vi "Acquire Every Image as Raw Data.vi"() -> ()   [LabVIEW 2023]
doc: "The Acquire Every Image as Raw Data example acquires images continuously and returns an array of the pixel data. This functionality can be useful for getting access to the raw data to stream it to disk in a binary format or pass it to a third-party processing function."
uses:
  <vilib>/vision/driver/IMAQdx.llb/IMAQdx Buffer Number Mode.ctl
  <vilib>/vision/driver/NI_Vision_Acquisition_Software.lvlib
  <resource>/objmgr/imaqdx.rc
panel:
  in  "Percent of Images Reserved by Driver":dbl=50.0
  in  "Overwrite Mode":u16(ring) items=["Get Oldest"=0, "Fail"=2, "Get Newest"=3]
  in  "Number of Images":i32=10
  out "Image Data Size (bytes)":i32
  out "Image Data":u8[](array[numeric])
  in  "Simulated Processing Delay (ms)":i32
  out "Images Missed":u32
  out "Images Behind":i32
  out "Processing Frame Rate":dbl
  in  "Camera Name":refnum<k21> caption="IMAQdx Session"
  out "Buffer Number":u32
  out "Acquired Frame Rate":dbl
  in  "Stop":bool
  # "Overview: Demonstrates how to acquire the raw data from a camera, which may be useful for streaming to disk or passing to third-party party image processing functions.\nRequirements: Vision Acquisition Software\nInstructions:\n1. Select the Camera Name\n2. Run the VI\n3. Increase the Simulated Processing Delay to see the effect on Images Behind and Images Missed when the acquisition loop isn't executed as quickly as the camera acquires images."
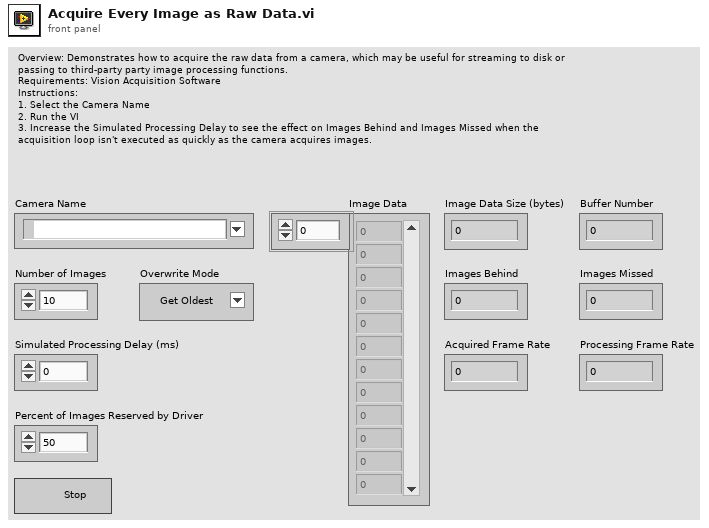
[diagram p1: front panel]
types:
  T1 = typedef "IMAQdx.ctl" = refnum<k21>
  T2 = typedef "NI_Vision_Acquisition_Software.lvlib/IMAQdx Buffer Number Mode.ctl" = enum32{"Next", "Last", "Buffer Number", "Every", "Last New"}
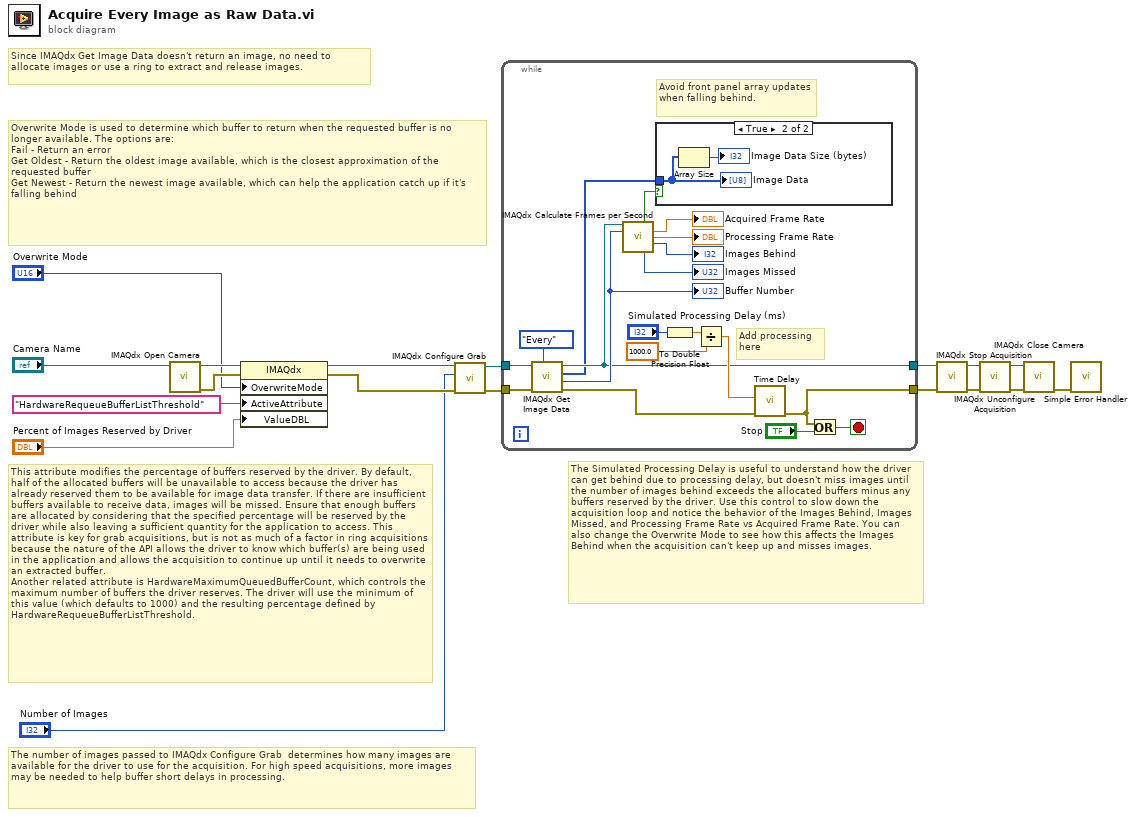
[diagram p0: block diagram]
diagram:
  # "The number of images passed to IMAQdx Configure Grab  determines how many images are available for the driver to use for the acquisition. For high speed acquisitions, more images may be needed to help buffer short delays in processing."
  # "This attribute modifies the percentage of buffers reserved by the driver. By default, half of the allocated buffers will be unavailable to access because the driver has already reserved them to be available for image data transfer. If there are insufficient buffers available to receive data, images will be missed. Ensure that enough buffers are allocated by considering that the specified percentage will be reserved by the driver while also leaving a sufficient quantity for the application to access. This attribute is key for grab acquisitions, but is not as much of a factor in ring acquisitions because the nature of the API allows the driver to know which buffer(s) are being used in the application and allows the acquisition to continue up until it needs to overwrite an extracted buffer.\nAnother related attribute is HardwareMaximumQueuedBufferCount, which controls the maximum number of buffers the driver reserves. The driver will use the minimum of this value (which defaults to 1000) and the resulting percentage defined by HardwareRequeueBufferListThreshold."
  # "The Simulated Processing Delay is useful to understand how the driver can get behind due to processing delay, but doesn't miss images until the number of images behind exceeds the allocated buffers minus any buffers reserved by the driver. Use this control to slow down the acquisition loop and notice the behavior of the Images Behind, Images Missed, and Processing Frame Rate vs Acquired Frame Rate. You can also change the Overwrite Mode to see how this affects the Images Behind when the acquisition can't keep up and misses images."
  # "Overwrite Mode is used to determine which buffer to return when the requested buffer is no longer available. The options are:\nFail - Return an error\nGet Oldest - Return the oldest image available, which is the closest approximation of the requested buffer\nGet Newest - Return the newest image available, which can help the application catch up if it's falling behind"
  # "Since IMAQdx Get Image Data doesn't return an image, no need to allocate images or use a ring to extract and release images."
  n1 = call <vilib>:"IMAQdx Open Camera.vi"("Session In"="Camera Name") -> ("error out"=w9:errorcluster, "Session Out"=w10:T1)  [unwired: 2 in, 7 out]
  n2 = property class="IMAQdx"(reference=w10, error in=w9, "OverwriteMode"="Overwrite Mode", "ActiveAttribute"="HardwareRequeueBufferListThreshold", "ValueDBL"="Percent of Images Reserved by Driver") -> (reference out=w8:T1, error out=w7:errorcluster)
  n3 = call <vilib>:"IMAQdx Configure Grab.vi"("error in"=w7, "Number of Buffers"="Number of Images", "Session In"=w8) -> ("error out"=w5:errorcluster, "Session Out"=w6:T1)  [unwired: 7 in]
  n4 = while {
    tunnel: [w24] -> w13
    tunnel: w5 -> [w27]
    tunnel: w6 -> [w28]
    tunnel: [w33] -> w12
    stop <- w37 stop-if-true
    # "Avoid front panel array updates when falling behind."
    # "Add processing here"
    n5 = call <vilib>:"IMAQdx Get Image Data.vi"("Buffer Number Mode (Next)"=IMAQdx_Buffer_Number_Mode."Every" ("Buffer Number Mode"), "error in"=w27, "Session In"=w28) -> ("error out"=w25:errorcluster, "Buffer Number Out"=w26:u32, "Image Data Array"=w23:u8[], "Session Out"=w24:T1)  [unwired: 1 in, 4 out]
    "Buffer Number" <- w26
    n6 = call <vilib>:"IMAQdx Calculate Frames per Second.vi"("Session In"=w24, "Buffer Number"=w26) -> ("Update Display"=w22:bool, "Acquired Frames per Second"=→"Acquired Frame Rate":dbl, "Processed Frames per Second"=→"Processing Frame Rate":dbl, "Images Behind"=→"Images Behind":i32, "Images Missed"=→"Images Missed":u32)  [unwired: 7 in, 2 out]
    n7 = case shown="True" w22 {
      tunnel: w23 -> [_ w38]
      frame False {
      }
      frame True {
        n8 = Array Size(array=w38) -> (size(s)=→"Image Data Size (bytes)":i32)
        "Image Data" <- w38
      }
    }
    n9 = To Double Precision Float(number="Simulated Processing Delay (ms)") -> (double precision float=w19:dbl)
    n10 = Divide(x=w19, y=1000.0) -> (x/y=w30:dbl)
    n11 = call "Time Delay"("error in (no error)"=w25, "Delay Time (s)"=w30) -> ("error out"=w33:errorcluster)  [unwired: 9 in]
    n12 = Or(x=w33, y="Stop") -> (x .or. y?=w37:bool)
  }
  n13 = call <vilib>:"IMAQdx Stop Acquisition.vi"("error in"=w12, "Session In"=w13) -> ("error out"=w15:errorcluster, "Session Out"=w16:T1)  [unwired: 8 out]
  n14 = call <vilib>:"IMAQdx Unconfigure Acquisition.vi"("error in"=w15, "Session In"=w16) -> ("error out"=w18:errorcluster, "Session Out"=w17:T1)  [unwired: 8 out]
  n15 = call <vilib>:"IMAQdx Close Camera.vi"("error in"=w18, "Session In"=w17) -> ("error out"=w11:errorcluster)  [unwired: 9 out]
  n16 = call <vilib>:"Simple Error Handler.vi"("error in (no error)"=w11) -> ()  [unwired: 4 in, 5 out]
